vi "main.vi"() -> ()   [LabVIEW 2017]
uses:
  libraryGcode/ControlGlobal/stateModeDevice.ctl
  libraryGcode/control/stateBoardFirmware.ctl
  libraryGcode/control/Queue/QueueCMDandPOS.ctl
  libraryGcode/control/Queue/TypeDataPOS.ctl
  libraryGcode/control/stateCmdUpdatePara.ctl
  C:/Users/annha/Desktop/Inverse Kinematic - demo/controls/Robot_definition.ctl
  LIN3D/Robot_testing_instructions.ctl
  libraryGcode/control/TypeFirmwareControl.ctl
  libraryGcode/ClassStringGcode/XuLyDataDisplay.lvclass
  <vilib>/Platform/TimedLoop/XDataNode/timing_clust.ctl
  <vilib>/Platform/TimedLoop/XDataNode/nitl_modes.ctl
  <vilib>/Platform/TimedLoop/XDataNode/wakeup.ctl
  libraryGcode/ClassParameter/stateLoop_View.ctl
  libraryGcode/ClassStringGcode/SelectMcode.ctl
  libraryGcode/ClassStringGcode/SelectGcode.ctl
  libraryGcode/variableGlobal/StartAutoandGcode.vi
  <vilib>/Platform/TimedLoop/XDataNode/XDataNode.xnode
  libraryGcode/LibraryGcode.lvlib
  <vilib>/Platform/TimedLoop/XDataNode/XDNodeRunTimeDep.lvlib
  <vilib>/picture/3D Picture Control/NI_3D Picture Control.lvlib
  libraryGcode/ClassParameter/ParameterConf.lvclass
panel:
  out "logical OR":bool
  in  "LeapJog":cluster{"X":sgl, "Y":sgl, "Z":sgl}
  out "degrees":cluster{"A":dbl, "B":dbl}
  out "error out 2":errorcluster
  out "error out":errorcluster
  out "data GET":string="w\n"
  out "POS":cluster{"X":dbl, "Y":dbl, "Z":dbl}
  out "STATE BOARD":T1=enum."Waiting"
  out "statusMode":T2=enum."Menu"
  in  "SwitchMode":bool
  in  "Exit Program":bool=TRUE
  in  "Tab Control":enum32{"Setting", "Auto", "Config", ""}(tab)
  out "Boolean":bool
  out "G2-G3 PARA":cluster{"X":dbl, "Y":dbl, "I":dbl, "J":dbl}
  in  "Send Gcode manual":T3
  in  "BUTTON CONTROL GCODE FILE":T4={"FILE"={"AddFile_ButtonSaveFile"=FALSE, "AddFile_ButtonDeleteLastLine"=FALSE, "AddFile_ButtonDeleteAll"=FALSE}, "MOTION"={"AddFile_ButtonGoHome"=TRUE, "AddFile_ButtonAddG1"=FALSE, "AddFile_ButtonAddG0"=FALSE}}
  in  "BUTTON CONTROL MANUAL":T5
  in  "PARA":cluster{"STEP":i16, "FEEDRATE":dbl}={"STEP"=10, "FEEDRATE"=500.0} {"FEEDRATE" min=0.0 max=10000.0 step=50.0; "STEP" min=0 max=90 step=2 format="%-1.0f"}
  in  "CONTROL PWM":T6={"SPIN"={"PWM"=55.0, "Control_buttonSpindle"=FALSE, "ButtonSPINDLE_ADD_FILE"=FALSE}, "FAN 1"={"Control_ButtonFan1"=FALSE, "PWM"=255.0, "AddFile_ButtonFan1"=FALSE}, "FAN 2"={"PWM"=0.0, "Control_ButtonFan2"=FALSE, "AddFile_ButtonFan2"=FALSE}, "FAN 3"={"PWM"=0.0, "Control_ButtonFan3"=FALSE, "AddFile_ButtonFan3"=FALSE}, "WAIT PIN"={"PIN INPUT"=55.0, "Control_ButtonWaitPin"=FALSE, "AddFile_ButtonWaitPin"=FALSE}, "SOLENOID"={"Control_ButtonSolenoid"=FALSE, "AddFile_ButtonSolenoid"=FALSE}} {"WAIT PIN"."PIN INPUT" min=55.0 max=58.0 step=1.0; "FAN 3"."PWM" min=0.0 max=255.0 step=5.0; "FAN 2"."PWM" min=0.0 max=255.0 step=5.0; "FAN 1"."PWM" min=0.0 max=255.0 step=10.0; "SPIN"."PWM" min=0.0 max=255.0 step=1.0}
  in  "Link Save File":path
  out "GCODE ADD":string="\r"
  in  "File to Cut":path
  in  "Start Auto":bool
  out "G-Code Array 2":string[](array[string])=["Loi khong ket noChua Chon File"]
  in  "RESET ERROR":bool
  in  "MAX FEEDRATE":T7={"DATA"={"X"=4000.0, "Y"=4000.0, "Z"=4000.0}, "Config_SetFeedrate"=FALSE}
  in  "MAX ACCEL":T8={"DATA"={"X"=5000.0, "Y"=5000.0, "Z"=500.0}, "Config_SetMaxACCEL"=FALSE}
  in  "STEPSIZE":T9={"DATA"={"X"=88.89, "Y"=88.89, "Z"=2133.33}, "Config_SetStepSize"=FALSE}
  in  "M204 Start AcceL":T10={"Config_SetSTARTACCEL"=FALSE, "data"={"P"=88.89, "R"=88.89, "T"=2133.33}}
  in  "Move":cluster{"X":dbl, "Y":dbl, "OK Button":bool}
  in  "Config_SaveEEPROM":bool
  out "output cluster 2":cluster{"angle 1":dbl, "angle 2":dbl, i32}
  out "3D Picture":refnum<vi>(3d-picture)
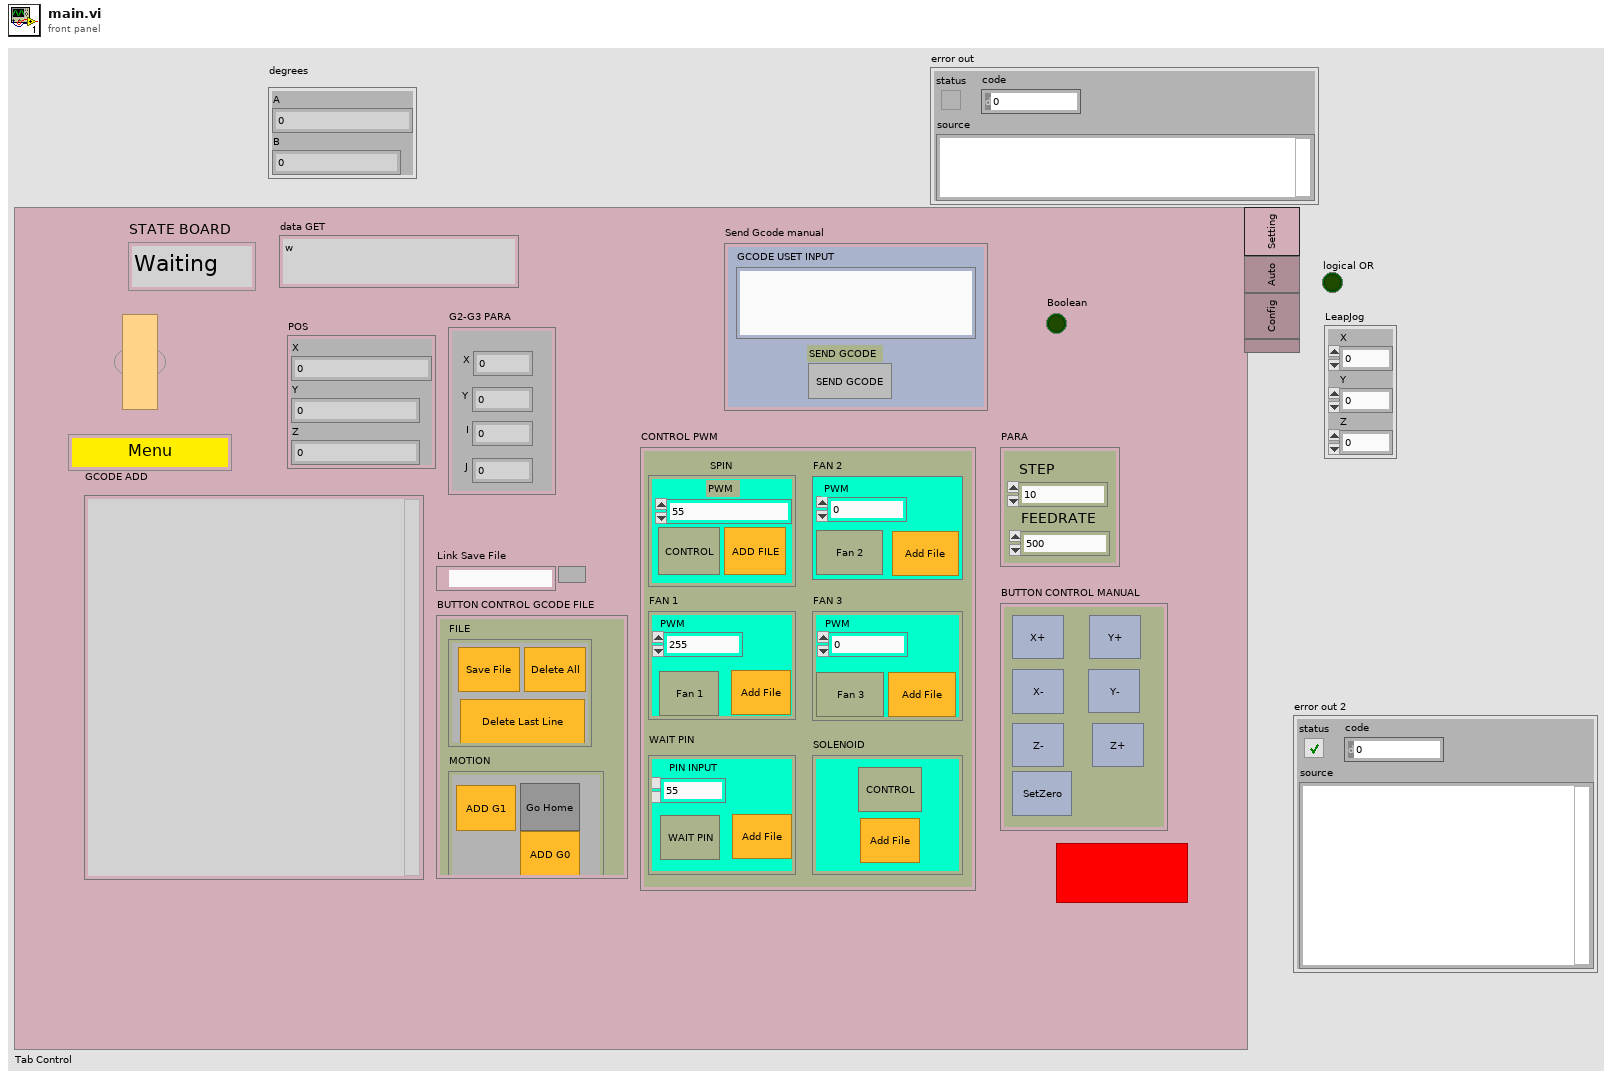
[diagram p1: front panel]
types:
  T1 = typedef "LibraryGcode.lvlib/stateBoardFirmware.ctl" = enum16{"Running", "Waiting", "Pos", "IDLE"}
  T2 = typedef "stateModeDevice.ctl" = enum16{"Auto", "Menu", "WaitAutoFinish", "Config", "initAuto"}
  T3 = cluster{"GCODE USET INPUT":string, "SEND GCODE":bool}
  T4 = cluster{"FILE":cluster{"AddFile_ButtonSaveFile":bool, "AddFile_ButtonDeleteLastLine":bool, "AddFile_ButtonDeleteAll":bool}, "MOTION":cluster{"AddFile_ButtonGoHome":bool, "AddFile_ButtonAddG1":bool, "AddFile_ButtonAddG0":bool}}
  T5 = cluster{"Control_ButtonX+":bool, "Control_ButtonX-":bool, "Control_ButtonY+":bool, "Control_ButtonY-":bool, "Control_ButtonZ+":bool, "Control_ButtonZ-":bool, "Control_ButtonSetZero":bool}
  T6 = cluster{"SPIN":cluster{"PWM":dbl, "Control_buttonSpindle":bool, "ButtonSPINDLE_ADD_FILE":bool}, "FAN 1":cluster{"Control_ButtonFan1":bool, "PWM":dbl, "AddFile_ButtonFan1":bool}, "FAN 2":cluster{"PWM":dbl, "Control_ButtonFan2":bool, "AddFile_ButtonFan2":bool}, "FAN 3":cluster{"PWM":dbl, "Control_ButtonFan3":bool, "AddFile_ButtonFan3":bool}, "WAIT PIN":cluster{"PIN INPUT":dbl, "Control_ButtonWaitPin":bool, "AddFile_ButtonWaitPin":bool}, "SOLENOID":cluster{"Control_ButtonSolenoid":bool, "AddFile_ButtonSolenoid":bool}}
  T7 = cluster{"DATA":cluster{"X":dbl, "Y":dbl, "Z":dbl}, "Config_SetFeedrate":bool}
  T8 = cluster{"DATA":cluster{"X":dbl, "Y":dbl, "Z":dbl}, "Config_SetMaxACCEL":bool}
  T9 = cluster{"DATA":cluster{"X":dbl, "Y":dbl, "Z":dbl}, "Config_SetStepSize":bool}
  T10 = cluster{"Config_SetSTARTACCEL":bool, "data":cluster{"P":dbl, "R":dbl, "T":dbl}}
  T11 = typedef "Robot_testing_instructions.ctl" = enum16{"idle", "Draw Robot", "Init 1 - Application", "Quit", "Close", "Error Handling", "Calculates"}
  T12 = typedef "Robot_definition.ctl" = cluster{"L2":sgl, "L3":sgl, "L1":sgl, "Base":sgl, "X0":sgl, "Z0":sgl}
  T13 = cluster{"Scene ref":refnum<vi>, "Arm 1 ref":refnum<vi>, "Arm 2 ref":refnum<vi>, "Arm 1 offset":cluster{"X":sgl, "Y":sgl, "Z":sgl}[], "Arm 2 offset":cluster{"X":sgl, "Y":sgl, "Z":sgl}[], "sand box":refnum<vi>, "Status":string, "A1":dbl, "A2":dbl, "Robot Definition":T12}
  T14 = typedef "LibraryGcode.lvlib/stateCmdUpdatePara.ctl" = enum16{"updatePos", "UpdateConfigAccel", "UpdateConfigFeed", "UpdateConfigUnit", "UpdateConfigStartAccel", "NoUpdate"}
  T15 = cluster{"Command":T14, "POS":cluster{"X":dbl, "Y":dbl, "Z":dbl}, "DEGREES":cluster{"X":dbl, "Y":dbl}}
  T16 = typedef "LibraryGcode.lvlib/QueueCMDandPOS.ctl" = cluster{"Serial Data Gcode":refnum<queue>, "cmdUpdateDisplay":refnum<queue>}
  T17 = typedef "LibraryGcode.lvlib/TypeFirmwareControl.ctl" = enum16{"ScaraMarlin", "CncMarlin", "Mk4Due"}
  T18 = typedef "XDNodeRunTimeDep.lvlib/timing_clust.ctl" = cluster{"Expected End [f-1]":u64, "Actual End [f-1]":u64, "Finished Late? [f-1]":bool, "Expected End [i-1]":u64, "Actual End [i-1]":u64, "Finished Late? [i-1]":bool, "Expected Start [i]":u64, "Actual Start [i]":u64, "Expected Start [f]":u64, "Actual Start [f]":u64, "Source Name":string, "Structure Name":string, "Period":i64, "Deadline":i64, "Offset":i64, "Start":i64, "Priority":i32, "Timeout":i32, "Mode":T19, "Wakeup Reason":T20, "Error":errorcluster, "Source Type":string, "Secondary Source Type":string, "Global End Time":u64, "Global Start Time":u64, "Frame Duration":u64, "Iteration Duration":u64, "Assigned CPU":i32, "I/O Scan Engine Mode":u32}
  T19 = typedef "XDNodeRunTimeDep.lvlib/nitl_modes.ctl" = enum32{"No Change", "Process missed periods, maintain original phase", "Discard missed periods, maintain original phase", "Process missed periods, ignore original phase", "Discard missed periods, ignore original phase"}
  T20 = typedef "XDNodeRunTimeDep.lvlib/wakeup.ctl" = enum32{"Normal", "Aborted", "Asynchronous wakeup", "Timing source error", "Timed loop error", "Timeout"}
  T21 = typedef "LibraryGcode.lvlib/XuLyDataDisplay.lvclass/SelectMcode.ctl" = enum16{"M204_SetStartingAcceleration", "M503_ReportSetting", "M500_SaveEprom", "M114_GetPosition", "M92_SetAxisStepPerUnit", "M17_EnableStep", "M18_DisableStep", "M80_PowerOn", "M81_PowerOff", "M112_EMGStop", "M118_SerialPrint", "M226_WaitforPinState", "M400_WaitFinishMove", "M203_SetMaxFeedRate", "M201_SetMaxACCEL", "M380_381_SetSoleNoid_On_Off", "M42_InitPin", "M42_PinControl", "M106_SetFan1", "M106_SetFan2", "M106_SetFan3", "M3_SetSpindle", "M5_OffSpindle", "M999_RestartStop"}
  T22 = typedef "LibraryGcode.lvlib/ParameterConf.lvclass/stateLoop_View.ctl" = enum16{"Running", "writeGlobal", "schedules500ms", "init", "End"}
  T23 = enum16{"Fan1", "Fan2", "Fan3", "PARA", "POS_DEGREE", "Solenoid", "Spindle", "TypeFirmware", "WaitPin", "MaxAcel", "MaxFeedrate", "MaxSize", "MaxStartAccel"}
  T24 = typedef "LibraryGcode.lvlib/XuLyDataDisplay.lvclass/SelectGcode.ctl" = enum16{"G0LinearMove", "G1XY", "G1LinearMove", "G2Arc", "G4Dwell", "G20InchUnit", "G21MilliUnit", "G28AutoHome", "G92SetPosition", "G90", "G91RelativePos", "JogX+", "JogX-", "JogY+", "JogY-", "JogZ+", "JogZ-", "sendGcodeString"}
  T25 = cluster{"SPIN":dbl, "FAN2":dbl, "FAN1":dbl, "FAN3":dbl, "WAIT PIN ":dbl}
  T26 = cluster{"PWM":dbl, "TypeFirmware":T17, "XYZ":cluster{"X":dbl, "Y":dbl, "Z":dbl}, "PARA":cluster{"STEP":i16, "FEEDRATE":dbl}, "DEGREES":cluster{"X":dbl, "Y":dbl}, "Solenoid":bool, "StartAccel":cluster{"P":dbl, "R":dbl, "T":dbl}}
  T27 = typedef "Robot_creation_loop_data.ctl" = cluster{"Robot Definition":T12, "Dispenser ref":refnum<vi>, "Arm 2 ref":refnum<vi>, "Arm 1 ref":refnum<vi>, "Base ref":refnum<vi>, "Scene ref":refnum<vi>, "Sand box ref":refnum<vi>, "Arm 1 Offset":cluster{"X":sgl, "Y":sgl, "Z":sgl}[], "Arm 2 Offset":cluster{"X":sgl, "Y":sgl, "Z":sgl}[], "Width":sgl}
  T28 = cluster{"error out":errorcluster, "error IO 2":errorcluster}
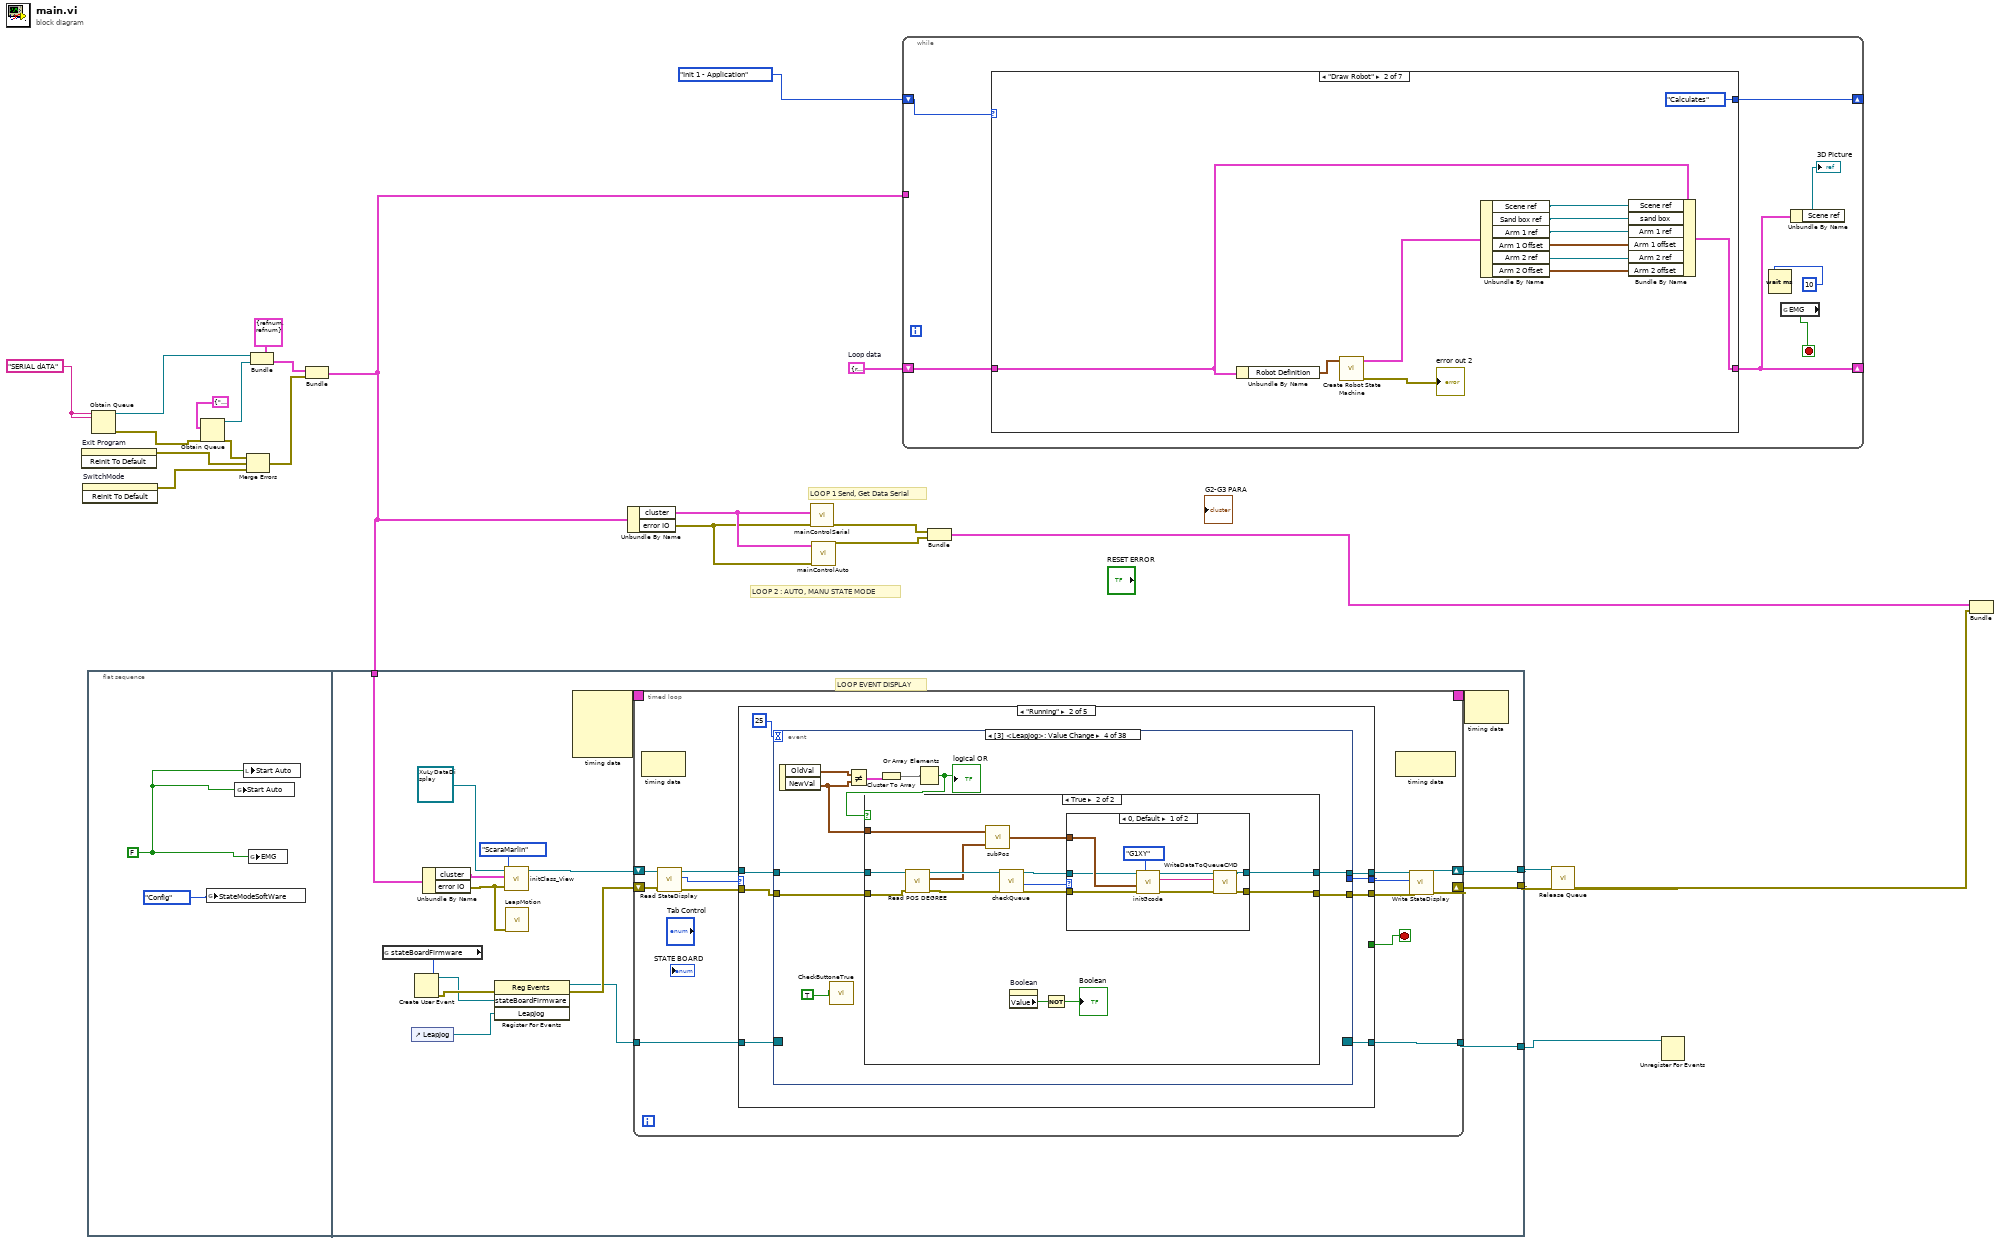
[diagram p0: block diagram]
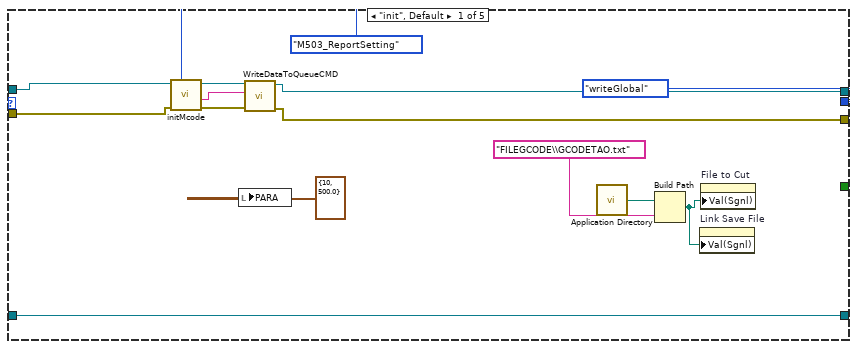
[diagram p2: hidden frame]
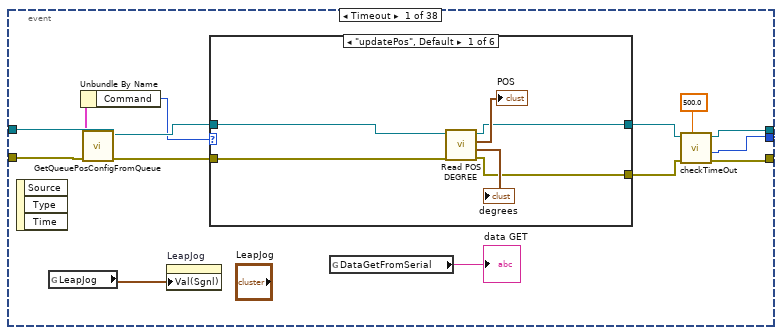
[diagram p3: hidden frame]
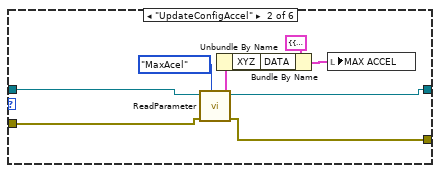
[diagram p4: hidden frame]
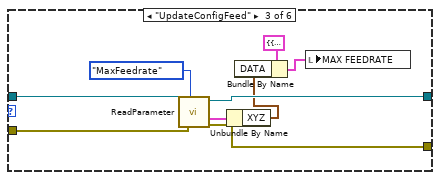
[diagram p5: hidden frame]
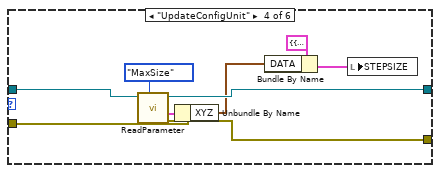
[diagram p6: hidden frame]
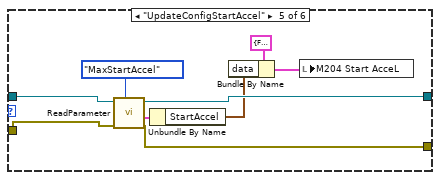
[diagram p7: hidden frame]
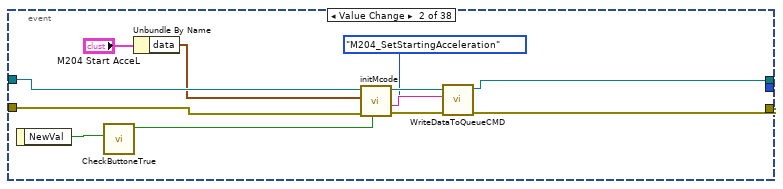
[diagram p9: hidden frame]
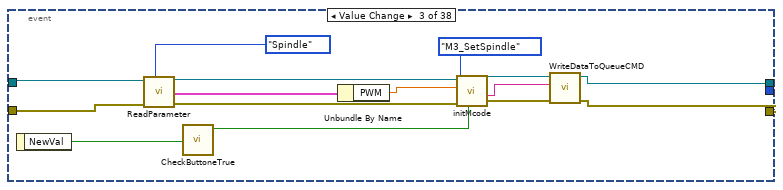
[diagram p10: hidden frame]
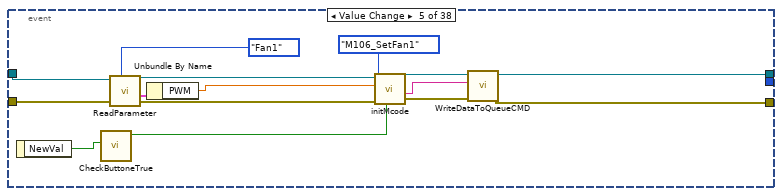
[diagram p13: hidden frame]
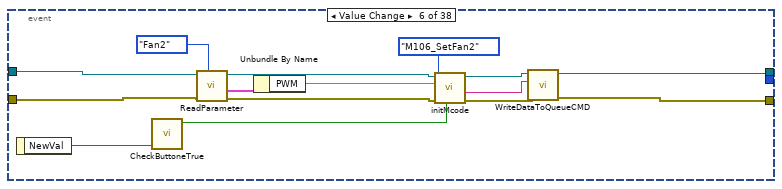
[diagram p14: hidden frame]
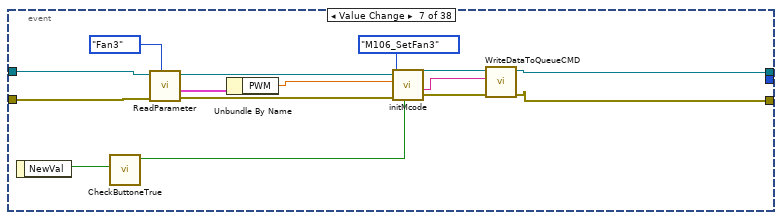
[diagram p15: hidden frame]
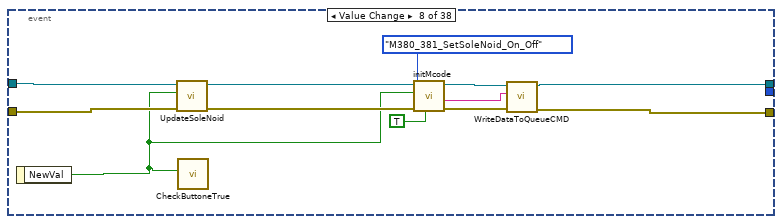
[diagram p16: hidden frame]
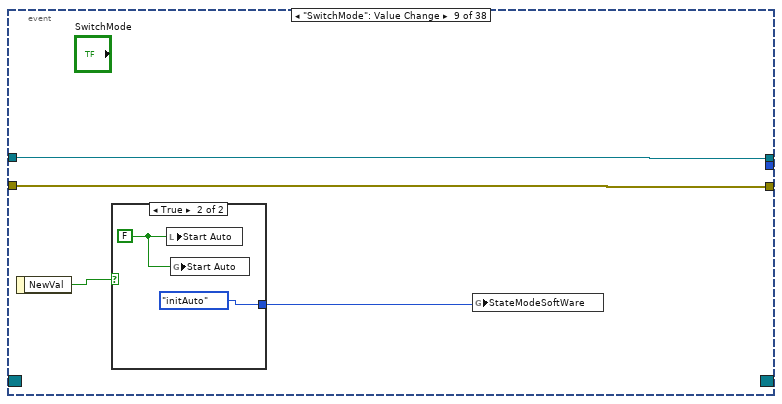
[diagram p17: hidden frame]
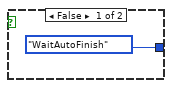
[diagram p18: hidden frame]
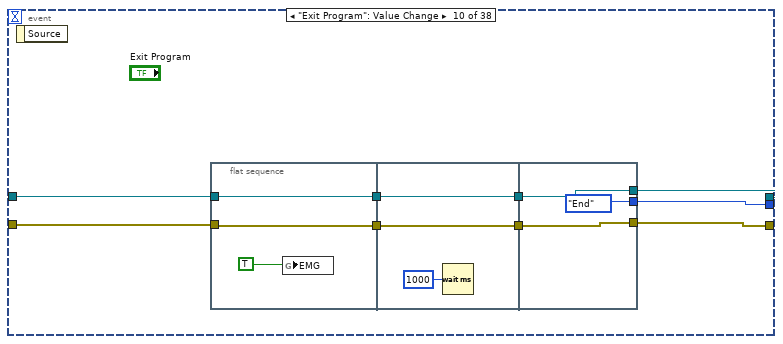
[diagram p19: hidden frame]
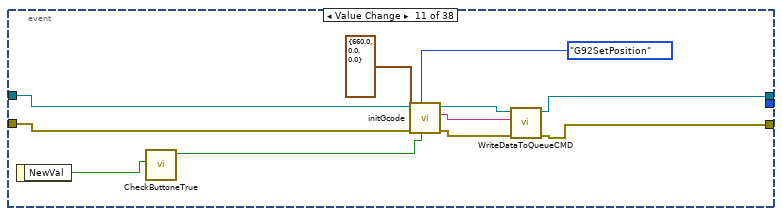
[diagram p20: hidden frame]
diagram:
  w9 = T13 {"Scene ref"=refnum, "Arm 1 ref"=refnum, "Arm 2 ref"=refnum, "Arm 1 offset"=[], "Arm 2 offset"=[], "sand box"=refnum, "Status"="", "A1"=43.0, "A2"=23.0, "Robot Definition"={"L2"=0.0, "L3"=0.0, "L1"=0.0, "Base"=0.0, "X0"=0.0, "Z0"=0.0}}  # Loop data
  w23 = "SERIAL dATA" ("name (unnamed)")
  # "LOOP 2 : AUTO, MANU STATE MODE"
  # "LOOP 1 Send, Get Data Serial"
  n1 = invoke on="Exit Program" class="Bool (strict)" method="Reinit To Default"() -> (error out=w21:errorcluster)  [unwired: 3 in, 2 out]
  n2 = invoke on="SwitchMode" class="Bool (strict)" method="Reinit To Default"() -> (error out=w22:errorcluster)  [unwired: 3 in, 2 out]
  n3 = flat-sequence {
    tunnel: [w42] -> w3
    tunnel: w11 -> [w41]
    tunnel: [w38] -> w4
    tunnel: [w28] -> w1
    frame #0 {
      w25 = FALSE ("Start Auto")
      n4 = global write "StartAutoandGcode.vi" "StateModeSoftWare"(stateModeDevice."Config" ("Enum")) -> ()
      n5 = global write "StartAutoandGcode.vi" "Start Auto"(w25) -> ()
      n6 = local write "Start Auto"(w25) -> ()
      n7 = global write "StartAutoandGcode.vi" "EMG"(w25) -> ()
    }
    frame #1 {
      # "LOOP EVENT DISPLAY"
      n8 = global read "StartAutoandGcode.vi" "stateBoardFirmware"() -> (w30:T1)
      n9 = control-ref of="LeapJog"() -> (w27:refnum<vi>)
      n10 = Create User Event(user event datatype=w30) -> (user event=w29:refnum<user-event>, error out=w32:errorcluster)  [unwired: 1 in]
      n11 = Unbundle By Name(w41) -> ("cluster"=w37:T16, "error IO"=w26:errorcluster)
      n12 = register-events(error in=w32, w29, w27) -> (reference out=w31:refnum<event-registration>, error out=w33:errorcluster)  [unwired: 1 in]
      n13 = call-dynamic "initClass_View.vi"("error in (no error)"=w26, "TypeFirmware"=TypeFirmwareControl."ScaraMarlin", "Queue Process"=w37, "XuLyDataDisplay in"=refnum<class "XuLyDataDisplay.lvclass"> refnum) -> ("XuLyDataDisplay out"=w35:refnum<class "XuLyDataDisplay.lvclass">)  [unwired: 6 in, 1 out]
      n14 = call "LeapMotion.vi"("Error In"=w26) -> ()  [unwired: 9 in, 2 out]
      n15 = node-c288() -> (w40:T18)  [unwired: 4 in]
      n16 = timed-loop {
        timing: w40 -> [_]
        timing-out: [_] -> w39
        shift-right: [w50] -> w38
        shift-left: w35 -> [w54]
        shift-right: [w49] -> w42
        shift-left: w33 -> [w52]
        tunnel: w31 -> [w44]
        tunnel: [w43] -> w28
        stop <- w55 stop-if-true
        n17 = node-c288() -> ()  [unwired: 1 in, 1 out]
        n18 = call-dynamic "Read StateDisplay.vi"("error in (no error)"=w52, "ParameterConf in"=w54) -> ("error out"=w51:errorcluster, "StateDisplay"=w47:T22, "ParameterConf out"=w53:refnum<class "XuLyDataDisplay.lvclass">)  [unwired: 7 in]
        n19 = case shown="\"Running\"" w47 {
          tunnel: w51 -> [w62 w72 w580 w592 w609]
          tunnel: [_ _ TRUE _ _] -> w55
          tunnel: [w61 w76 w580 w590 w606] -> w48
          tunnel: w53 -> [w66 w78 w579 w593 w610]
          tunnel: [w63 w74 w579 w591 w607] -> w45
          tunnel: [stateLoop_View."writeGlobal" ("StateDisplay") w77 stateLoop_View."init" ("StateDisplay") stateLoop_View."schedules500ms" ("StateDisplay") stateLoop_View."Running" ("StateDisplay")] -> w46
          tunnel: w44 -> [w58 w75 w577 w582 w604]
          tunnel: [w58 w73 w577 w582 w604] -> w43
          frame "init", Default {
            n20 = call-dynamic "initMcode.vi"("error in (no error)"=w62, "mCode"=SelectMcode."M503_ReportSetting", "XuLyDataDisplay in"=w66) -> ("error out"=w60:errorcluster, "McodeOut"=w64:string, "XuLyDataDisplay out"=w65:refnum<class "XuLyDataDisplay.lvclass">)  [unwired: 6 in]
            n21 = local write "PARA"(cluster{"STEP":i16, "FEEDRATE":dbl} {"STEP"=10, "FEEDRATE"=500.0} ("PARA")) -> ()
            n22 = call-dynamic "WriteDataToQueueCMD.vi"("error in (no error)"=w60, "DataIn"=w64, "ParameterConf in"=w65) -> ("error out"=w61:errorcluster, "ParameterConf out"=w63:refnum<class "XuLyDataDisplay.lvclass">)  [unwired: 7 in]
            n23 = call <vilib>:"Application Directory.vi"() -> ("Application Directory"=w69:path)
            n24 = Build Path(base path=w69, name or relative path="FILEGCODE\\GCODETAO.txt") -> (appended path=w71:path)
            n25 = property on="Link Save File" class="Path"("Val(Sgnl)"=w71) -> ()  [unwired: 2 in, 2 out]
            n26 = property on="File to Cut" class="Path"("Val(Sgnl)"=w71) -> ()  [unwired: 2 in, 2 out]
          }
          frame "Running" {
            n27 = event shown="[3] <LeapJog>: Value Change" {
              selector: w75 -> [_ _ _ _ _ _ _ _ _ _ _ _ _ _ _ _ _ _ _ _ _ _ _ _ _ _ _ _ _ _ _ _ _ _ w536 _ _ _]
              dyn-events: [_ _ _ _ _ _ _ _ _ _ _ _ _ _ _ _ _ _ _ _ _ _ _ _ _ _ _ _ _ _ _ _ _ _ w536 _ _ _] -> w73
              timeout: 25 -> [_ _ _ _ _ _ _ _ _ _ _ _ _ _ _ _ _ _ _ _ _ _ _ _ _ _ _ _ _ _ _ _ _ _ _ _ _ _]
              tunnel: w72 -> [w92 w142 w162 w168 w213 w228 w244 w256 w261 w267 w290 w295 w300 w312 w328 w337 w351 w364 w370 w382 w395 w401 w420 w435 w446 w463 w478 w484 w488 w490 w499 w511 w521 w533 w544 w554 w560 w570]
              tunnel: [w84 w145 w153 w167 w209 w222 w238 w250 w261 w266 w285 w295 w298 w314 w323 w339 w348 w359 w370 w374 w395 w400 w407 w423 w438 w453 w466 w481 w488 w491 w502 w505 w522 w531 w540 w547 w557 w569] -> w76
              tunnel: w78 -> [w93 w148 w163 w170 w214 w229 w243 w257 w260 w270 w291 w294 w301 w316 w329 w342 w352 w366 w369 w383 w396 w402 w421 w436 w447 w464 w479 w485 w487 w493 w501 w512 w524 w534 w545 w555 w561 w571]
              tunnel: [w85 w146 w154 w169 w210 w223 w239 w253 w260 w273 w286 w294 w296 w313 w324 w340 w349 w357 w369 w373 w396 w397 w408 w424 w439 w454 w467 w482 w487 w489 w494 w506 w523 w532 w541 w548 w558 w567] -> w74
              tunnel: [w82 _ _ _ _ _ _ _ _ w265 _ _ _ _ _ _ _ _ _ _ stateLoop_View."writeGlobal" ("StateDisplay") _ _ _ _ _ _ _ _ _ _ _ _ _ _ _ _ _] -> w77
              event Timeout {
                n28 = event-data() -> ()  [unwired: 1 in, 3 out]
                n29 = global read "StartAutoandGcode.vi" "LeapJog"() -> (w80:cluster{"X":sgl, "Y":sgl, "Z":sgl})
                n30 = call-dynamic "GetQueuePosConfigFromQueue.vi"("error in (no error)"=w92, "ParameterConf in"=w93) -> ("error out"=w89:errorcluster, "element"=w91:T15, "ParameterConf out"=w90:refnum<class "XuLyDataDisplay.lvclass">)  [unwired: 7 in]
                n31 = Unbundle By Name(w91) -> ("Command"=w81:T14)
                n32 = property on="LeapJog" class="Clust (strict)"("Val(Sgnl)"=w80) -> ()  [unwired: 2 in, 2 out]
                n33 = case shown="\"updatePos\", Default" w81 {
                  tunnel: [w95 w108 w115 w125 w134 w137] -> w87
                  tunnel: w90 -> [w97 w107 w117 w118 w130 w137]
                  tunnel: [w94 w105 w114 w124 w133 w136] -> w86
                  tunnel: w89 -> [w96 w106 w116 w126 w135 w136]
                  frame "updatePos", Default {
                    n34 = call-dynamic "Read POS DEGREE.vi"("error in (no error)"=w96, "ParameterConf in"=w97) -> ("error out"=w94:errorcluster, "DEGREES"=→"degrees":cluster{"X":dbl, "Y":dbl}, "POS"=→"POS":cluster{"X":dbl, "Y":dbl, "Z":dbl}, "ParameterConf out"=w95:refnum<class "XuLyDataDisplay.lvclass">)  [unwired: 6 in]
                  }
                  frame "UpdateConfigAccel" {
                    n35 = call-dynamic "ReadParameter.vi"("ParameterConf in"=w107, "error in (no error)"=w106, "Parameter"=T23."MaxAcel") -> ("ParameterConf out"=w108:refnum<class "XuLyDataDisplay.lvclass">, "DataOutClust"=w101:T26, "error out"=w105:errorcluster)  [unwired: 4 in, 1 out]
                    n36 = Unbundle By Name(w101) -> ("XYZ"=w100:cluster{"X":dbl, "Y":dbl, "Z":dbl})
                    n37 = Bundle By Name(cluster=T8 {"DATA"={"X"=355.0, "Y"=355.0, "Z"=2133.0}, "Config_SetMaxACCEL"=FALSE} ("MAX ACCEL"), "DATA"=w100) -> (w103:T8)
                    n38 = local write "MAX ACCEL"(w103) -> ()
                  }
                  frame "UpdateConfigFeed" {
                    n39 = call-dynamic "ReadParameter.vi"("ParameterConf in"=w117, "error in (no error)"=w116, "Parameter"=T23."MaxFeedrate") -> ("ParameterConf out"=w115:refnum<class "XuLyDataDisplay.lvclass">, "DataOutClust"=w110:T26, "error out"=w114:errorcluster)  [unwired: 4 in, 1 out]
                    n40 = Unbundle By Name(w110) -> ("XYZ"=w109:cluster{"X":dbl, "Y":dbl, "Z":dbl})
                    n41 = Bundle By Name(cluster=T9 {"DATA"={"X"=355.56, "Y"=355.56, "Z"=2133.33}, "Config_SetStepSize"=FALSE} ("STEPSIZE"), "DATA"=w109) -> (w112:T9)
                    n42 = local write "MAX FEEDRATE"(w112) -> ()
                  }
                  frame "UpdateConfigUnit" {
                    n43 = call-dynamic "ReadParameter.vi"("ParameterConf in"=w118, "error in (no error)"=w126, "Parameter"=T23."MaxSize") -> ("ParameterConf out"=w125:refnum<class "XuLyDataDisplay.lvclass">, "DataOutClust"=w120:T26, "error out"=w124:errorcluster)  [unwired: 4 in, 1 out]
                    n44 = Unbundle By Name(w120) -> ("XYZ"=w119:cluster{"X":dbl, "Y":dbl, "Z":dbl})
                    n45 = Bundle By Name(cluster=T7 {"DATA"={"X"=150000.0, "Y"=150000.0, "Z"=10000.0}, "Config_SetFeedrate"=FALSE} ("MAX FEEDRATE"), "DATA"=w119) -> (w122:T7)
                    n46 = local write "STEPSIZE"(w122) -> ()
                  }
                  frame "UpdateConfigStartAccel" {
                    n47 = call-dynamic "ReadParameter.vi"("ParameterConf in"=w130, "error in (no error)"=w135, "Parameter"=T23."MaxStartAccel") -> ("ParameterConf out"=w134:refnum<class "XuLyDataDisplay.lvclass">, "DataOutClust"=w128:T26, "error out"=w133:errorcluster)  [unwired: 4 in, 1 out]
                    n48 = Unbundle By Name(w128) -> ("StartAccel"=w127:cluster{"P":dbl, "R":dbl, "T":dbl})
                    n49 = Bundle By Name(cluster=T10 {"Config_SetSTARTACCEL"=FALSE, "data"={"P"=355.56, "R"=355.56, "T"=2133.33}} ("M204 Start AcceL"), "data"=w127) -> (w131:T10)
                    n50 = local write "M204 Start AcceL"(w131) -> ()
                  }
                  frame "NoUpdate" {
                  }
                }
                n51 = global read "StartAutoandGcode.vi" "DataGetFromSerial"() -> (→"data GET":string)
                n52 = call-dynamic "checkTimeOut.vi"("error in (no error)"=w86, "Time"=500.0, "ParameterConf in"=w87) -> ("error out"=w84:errorcluster, "stateDisplay"=w82:T22, "ParameterConf out"=w85:refnum<class "XuLyDataDisplay.lvclass">)  [unwired: 5 in, 1 out]
              }
              event "M204 Start AcceL.Config_SetSTARTACCEL": Value Change {
                n53 = event-data() -> ("NewVal"=w149:bool)  [unwired: 1 in]
                n54 = call "CheckButtoneTrue.vi"("IN"=w149) -> ("OUT"=w138:bool)  [unwired: 10 in]
                n55 = Unbundle By Name("M204 Start AcceL") -> ("data"=w140:cluster{"P":dbl, "R":dbl, "T":dbl})
                n56 = call-dynamic "initMcode.vi"("CheckMenu"=w138, "error in (no error)"=w142, "mCode"=SelectMcode."M204_SetStartingAcceleration", "DataVariant"=w140, "XuLyDataDisplay in"=w148) -> ("error out"=w144:errorcluster, "McodeOut"=w143:string, "XuLyDataDisplay out"=w147:refnum<class "XuLyDataDisplay.lvclass">)  [unwired: 4 in]
                n57 = call-dynamic "WriteDataToQueueCMD.vi"("error in (no error)"=w144, "DataIn"=w143, "ParameterConf in"=w147) -> ("error out"=w145:errorcluster, "ParameterConf out"=w146:refnum<class "XuLyDataDisplay.lvclass">)  [unwired: 7 in]
              }
              event "CONTROL PWM.SPIN.Control_buttonSpindle": Value Change {
                n58 = event-data() -> ("NewVal"=w164:bool)  [unwired: 1 in]
                n59 = call-dynamic "ReadParameter.vi"("ParameterConf in"=w163, "error in (no error)"=w162, "Parameter"=T23."Spindle") -> ("ParameterConf out"=w160:refnum<class "XuLyDataDisplay.lvclass">, "DataOutClust"=w152:T26, "error out"=w159:errorcluster)  [unwired: 4 in, 1 out]
                n60 = call "CheckButtoneTrue.vi"("IN"=w164) -> ("OUT"=w157:bool)  [unwired: 10 in]
                n61 = Unbundle By Name(w152) -> ("PWM"=w151:dbl)
                n62 = call-dynamic "initMcode.vi"("CheckMenu"=w157, "error in (no error)"=w159, "mCode"=SelectMcode."M3_SetSpindle", "DataVariant"=w151, "XuLyDataDisplay in"=w160) -> ("error out"=w158:errorcluster, "McodeOut"=w156:string, "XuLyDataDisplay out"=w161:refnum<class "XuLyDataDisplay.lvclass">)  [unwired: 4 in]
                n63 = call-dynamic "WriteDataToQueueCMD.vi"("error in (no error)"=w158, "DataIn"=w156, "ParameterConf in"=w161) -> ("error out"=w153:errorcluster, "ParameterConf out"=w154:refnum<class "XuLyDataDisplay.lvclass">)  [unwired: 7 in]
              }
              event Value Change {
                n64 = event-data() -> ("OldVal"=w173:cluster{"X":sgl, "Y":sgl, "Z":sgl}, "NewVal"=w165:cluster{"X":sgl, "Y":sgl, "Z":sgl})  [unwired: 1 in]
                n65 = call "CheckButtoneTrue.vi"("IN"=TRUE) -> ()  [unwired: 10 in, 1 out]
                n66 = Not Equal?(x=w173, y=w165) -> (x != y?=w172:cluster{"X":bool, "Y":bool, "Z":bool})
                n67 = Cluster To Array(cluster=w172) -> (array=w171:bool[])
                n68 = Or Array Elements(Boolean array=w171) -> (logical OR=w166:bool)
                "logical OR" <- w166
                n69 = case shown="True" w166 {
                  tunnel: w170 -> [w176 w189]
                  tunnel: [w176 w182] -> w169
                  tunnel: w168 -> [w175 w187]
                  tunnel: [w175 w181] -> w167
                  tunnel: w165 -> [_ w185]
                  frame False {
                  }
                  frame True {
                    n70 = call-dynamic "Read POS DEGREE.vi"("error in (no error)"=w187, "ParameterConf in"=w189) -> ("error out"=w183:errorcluster, "POS"=w186:cluster{"X":dbl, "Y":dbl, "Z":dbl}, "ParameterConf out"=w188:refnum<class "XuLyDataDisplay.lvclass">)  [unwired: 6 in, 1 out]
                    n71 = call "subPos.vi"("POS"=w186, "NewVal"=w185) -> ("PosSetG92"=w184:cluster{"X":dbl, "Y":dbl, "Z":dbl})
                    n72 = call-dynamic "checkQueue.vi"("ParameterConf in"=w188) -> ("Numeric"=w177:i16, "ParameterConf out"=w178:refnum<class "XuLyDataDisplay.lvclass">)  [unwired: 8 in, 1 out]
                    n73 = property on="Boolean" class="Bool (strict)"() -> ("Value"=w179:bool)  [unwired: 2 in, 2 out]
                    n74 = Not(x=w179) -> (.not. x?=→"Boolean":bool)
                    n75 = case shown="0, Default" w177 {
                      tunnel: w184 -> [w196 _]
                      tunnel: w183 -> [w195 w199]
                      tunnel: [w194 w200] -> w182
                      tunnel: [w191 w199] -> w181
                      tunnel: w178 -> [w190 w200]
                      frame 0, Default {
                        n76 = call-dynamic "initGcode.vi"("gCode"=SelectGcode."G1XY", "error in (no error)"=w195, "PosSetG92"=w196, "XuLyDataDisplay in"=w190) -> ("error out"=w192:errorcluster, "GcodeString Out"=w193:string, "XuLyDataDisplay out"=w198:refnum<class "XuLyDataDisplay.lvclass">)  [unwired: 5 in]
                        n77 = call-dynamic "WriteDataToQueueCMD.vi"("error in (no error)"=w192, "DataIn"=w193, "ParameterConf in"=w198) -> ("error out"=w191:errorcluster, "ParameterConf out"=w194:refnum<class "XuLyDataDisplay.lvclass">)  [unwired: 7 in]
                      }
                      frame 1 {
                      }
                    }
                  }
                }
              }
              event "CONTROL PWM.FAN 1.Control_ButtonFan1": Value Change {
                n78 = event-data() -> ("NewVal"=w215:bool)  [unwired: 1 in]
                n79 = call "CheckButtoneTrue.vi"("IN"=w215) -> ("OUT"=w204:bool)  [unwired: 10 in]
                n80 = call-dynamic "ReadParameter.vi"("ParameterConf in"=w214, "error in (no error)"=w213, "Parameter"=T23."Fan1") -> ("ParameterConf out"=w212:refnum<class "XuLyDataDisplay.lvclass">, "DataOutClust"=w203:T26, "error out"=w208:errorcluster)  [unwired: 4 in, 1 out]
                n81 = Unbundle By Name(w203) -> ("PWM"=w202:dbl)
                n82 = call-dynamic "initMcode.vi"("CheckMenu"=w204, "error in (no error)"=w208, "mCode"=SelectMcode."M106_SetFan1", "DataVariant"=w202, "XuLyDataDisplay in"=w212) -> ("error out"=w206:errorcluster, "McodeOut"=w205:string, "XuLyDataDisplay out"=w211:refnum<class "XuLyDataDisplay.lvclass">)  [unwired: 4 in]
                n83 = call-dynamic "WriteDataToQueueCMD.vi"("error in (no error)"=w206, "DataIn"=w205, "ParameterConf in"=w211) -> ("error out"=w209:errorcluster, "ParameterConf out"=w210:refnum<class "XuLyDataDisplay.lvclass">)  [unwired: 7 in]
              }
              event "CONTROL PWM.FAN 2.Control_ButtonFan2": Value Change {
                n84 = event-data() -> ("NewVal"=w230:bool)  [unwired: 1 in]
                n85 = call "CheckButtoneTrue.vi"("IN"=w230) -> ("OUT"=w220:bool)  [unwired: 10 in]
                n86 = call-dynamic "ReadParameter.vi"("ParameterConf in"=w229, "error in (no error)"=w228, "Parameter"=T23."Fan2") -> ("ParameterConf out"=w227:refnum<class "XuLyDataDisplay.lvclass">, "DataOutClust"=w218:T26, "error out"=w221:errorcluster)  [unwired: 4 in, 1 out]
                n87 = Unbundle By Name(w218) -> ("PWM"=w216:dbl)
                n88 = call-dynamic "initMcode.vi"("CheckMenu"=w220, "error in (no error)"=w221, "mCode"=SelectMcode."M106_SetFan2", "DataVariant"=w216, "XuLyDataDisplay in"=w227) -> ("error out"=w224:errorcluster, "McodeOut"=w226:string, "XuLyDataDisplay out"=w225:refnum<class "XuLyDataDisplay.lvclass">)  [unwired: 4 in]
                n89 = call-dynamic "WriteDataToQueueCMD.vi"("error in (no error)"=w224, "DataIn"=w226, "ParameterConf in"=w225) -> ("error out"=w222:errorcluster, "ParameterConf out"=w223:refnum<class "XuLyDataDisplay.lvclass">)  [unwired: 7 in]
              }
              event "CONTROL PWM.FAN 3.Control_ButtonFan3": Value Change {
                n90 = event-data() -> ("NewVal"=w245:bool)  [unwired: 1 in]
                n91 = call "CheckButtoneTrue.vi"("IN"=w245) -> ("OUT"=w234:bool)  [unwired: 10 in]
                n92 = call-dynamic "ReadParameter.vi"("ParameterConf in"=w243, "error in (no error)"=w244, "Parameter"=T23."Fan3") -> ("ParameterConf out"=w242:refnum<class "XuLyDataDisplay.lvclass">, "DataOutClust"=w232:T26, "error out"=w236:errorcluster)  [unwired: 4 in, 1 out]
                n93 = Unbundle By Name(w232) -> ("PWM"=w231:dbl)
                n94 = call-dynamic "initMcode.vi"("CheckMenu"=w234, "error in (no error)"=w236, "mCode"=SelectMcode."M106_SetFan3", "DataVariant"=w231, "XuLyDataDisplay in"=w242) -> ("error out"=w237:errorcluster, "McodeOut"=w241:string, "XuLyDataDisplay out"=w240:refnum<class "XuLyDataDisplay.lvclass">)  [unwired: 4 in]
                n95 = call-dynamic "WriteDataToQueueCMD.vi"("error in (no error)"=w237, "DataIn"=w241, "ParameterConf in"=w240) -> ("error out"=w238:errorcluster, "ParameterConf out"=w239:refnum<class "XuLyDataDisplay.lvclass">)  [unwired: 7 in]
              }
              event "CONTROL PWM.SOLENOID.Control_ButtonSolenoid": Value Change {
                n96 = event-data() -> ("NewVal"=w247:bool)  [unwired: 1 in]
                n97 = call-dynamic "UpdateSoleNoid.vi"("error in (no error)"=w256, "Boolean"=w247, "ParameterConf in"=w257) -> ("error out"=w252:errorcluster, "ParameterConf out"=w255:refnum<class "XuLyDataDisplay.lvclass">)  [unwired: 7 in]
                n98 = call "CheckButtoneTrue.vi"("IN"=w247) -> ()  [unwired: 10 in, 1 out]
                n99 = call-dynamic "initMcode.vi"("CheckMenu"=TRUE, "error in (no error)"=w252, "mCode"=SelectMcode."M380_381_SetSoleNoid_On_Off", "DataVariant"=w247, "XuLyDataDisplay in"=w255) -> ("error out"=w251:errorcluster, "McodeOut"=w248:string, "XuLyDataDisplay out"=w254:refnum<class "XuLyDataDisplay.lvclass">)  [unwired: 4 in]
                n100 = call-dynamic "WriteDataToQueueCMD.vi"("error in (no error)"=w251, "DataIn"=w248, "ParameterConf in"=w254) -> ("error out"=w250:errorcluster, "ParameterConf out"=w253:refnum<class "XuLyDataDisplay.lvclass">)  [unwired: 7 in]
              }
              event "SwitchMode": Value Change {
                n101 = event-data() -> ("NewVal"=w259:bool)  [unwired: 1 in]
                n102 = case shown="True" w259 {
                  tunnel: [stateModeDevice."WaitAutoFinish" ("Enum") stateModeDevice."initAuto" ("Enum")] -> w258
                  frame False {
                  }
                  frame True {
                    w263 = FALSE ("Start Auto")
                    n103 = local write "Start Auto"(w263) -> ()
                    n104 = global write "StartAutoandGcode.vi" "Start Auto"(w263) -> ()
                  }
                }
                n105 = global write "StartAutoandGcode.vi" "StateModeSoftWare"(w258) -> ()
              }
              event "Exit Program": Value Change {
                n106 = event-data() -> ()  [unwired: 1 in, 1 out]
                n107 = flat-sequence {
                  tunnel: [w276] -> w271
                  tunnel: w270 -> [w276]
                  tunnel: [w275] -> w268
                  tunnel: w267 -> [w275]
                  tunnel: [w278] -> w272
                  tunnel: w271 -> [w278]
                  tunnel: [w277] -> w269
                  tunnel: w268 -> [w277]
                  tunnel: [w282] -> w273
                  tunnel: w272 -> [w282]
                  tunnel: [w281] -> w266
                  tunnel: w269 -> [w281]
                  tunnel: [stateLoop_View."End" ("StateDisplay")] -> w265
                  frame #0 {
                    n108 = global write "StartAutoandGcode.vi" "EMG"(TRUE ("EMG1")) -> ()
                  }
                  frame #1 {
                    n109 = Wait (ms)(milliseconds to wait=u32 1000) -> ()  [unwired: 1 out]
                  }
                  frame #2 {
                  }
                }
              }
              event "BUTTON CONTROL MANUAL.Control_ButtonSetZero": Value Change {
                n110 = event-data() -> ("NewVal"=w284:bool)  [unwired: 1 in]
                n111 = call "CheckButtoneTrue.vi"("IN"=w284) -> ("OUT"=w283:bool)  [unwired: 10 in]
                n112 = call-dynamic "initGcode.vi"("Che Do"=w283, "gCode"=SelectGcode."G92SetPosition", "error in (no error)"=w290, "PosSetG92"=cluster{"X":dbl, "Y":dbl, "Z":dbl} {"X"=660.0, "Y"=0.0, "Z"=0.0}, "XuLyDataDisplay in"=w291) -> ("error out"=w287:errorcluster, "GcodeString Out"=w288:string, "XuLyDataDisplay out"=w289:refnum<class "XuLyDataDisplay.lvclass">)  [unwired: 4 in]
                n113 = call-dynamic "WriteDataToQueueCMD.vi"("error in (no error)"=w287, "DataIn"=w288, "ParameterConf in"=w289) -> ("error out"=w285:errorcluster, "ParameterConf out"=w286:refnum<class "XuLyDataDisplay.lvclass">)  [unwired: 7 in]
              }
              event "Tab Control": Value Change {
                n114 = event-data() -> ()  [unwired: 1 in, 1 out]
              }
              event "BUTTON CONTROL MANUAL.Control_ButtonX+": Value Change {
                n115 = event-data() -> ("NewVal"=w305:bool)  [unwired: 1 in]
                n116 = call "CheckButtoneTrue.vi"("IN"=w305) -> ("OUT"=w299:bool)  [unwired: 10 in]
                n117 = call-dynamic "initGcode.vi"("Che Do"=w299, "gCode"=SelectGcode."JogX+", "error in (no error)"=w300, "XuLyDataDisplay in"=w301) -> ("error out"=w303:errorcluster, "GcodeString Out"=w297:string, "XuLyDataDisplay out"=w304:refnum<class "XuLyDataDisplay.lvclass">)  [unwired: 5 in]
                n118 = call-dynamic "WriteDataToQueueCMD.vi"("error in (no error)"=w303, "DataIn"=w297, "ParameterConf in"=w304) -> ("error out"=w298:errorcluster, "ParameterConf out"=w296:refnum<class "XuLyDataDisplay.lvclass">)  [unwired: 7 in]
              }
              event "MAX FEEDRATE.Config_SetFeedrate": Value Change {
                n119 = event-data() -> ("NewVal"=w318:bool)  [unwired: 1 in]
                n120 = call "CheckButtoneTrue.vi"("IN"=w318) -> ("OUT"=w315:bool)  [unwired: 10 in]
                n121 = Unbundle By Name("MAX FEEDRATE") -> ("DATA"=w306:cluster{"X":dbl, "Y":dbl, "Z":dbl})
                n122 = To Variant(anything=w306) -> (Variant=w309:variant)
                n123 = call-dynamic "initMcode.vi"("CheckMenu"=w315, "error in (no error)"=w312, "mCode"=SelectMcode."M203_SetMaxFeedRate", "DataVariant"=w309, "XuLyDataDisplay in"=w316) -> ("error out"=w311:errorcluster, "McodeOut"=w308:string, "XuLyDataDisplay out"=w317:refnum<class "XuLyDataDisplay.lvclass">)  [unwired: 4 in]
                n124 = call-dynamic "WriteDataToQueueCMD.vi"("error in (no error)"=w311, "DataIn"=w308, "ParameterConf in"=w317) -> ("error out"=w314:errorcluster, "ParameterConf out"=w313:refnum<class "XuLyDataDisplay.lvclass">)  [unwired: 7 in]
              }
              event "MAX ACCEL.Config_SetMaxACCEL": Value Change {
                n125 = event-data() -> ("NewVal"=w331:bool)  [unwired: 1 in]
                n126 = call "CheckButtoneTrue.vi"("IN"=w331) -> ("OUT"=w330:bool)  [unwired: 10 in]
                n127 = Unbundle By Name("MAX ACCEL") -> ("DATA"=w320:cluster{"X":dbl, "Y":dbl, "Z":dbl})
                n128 = To Variant(anything=w320) -> (Variant=w322:variant)
                n129 = call-dynamic "initMcode.vi"("CheckMenu"=w330, "error in (no error)"=w328, "mCode"=SelectMcode."M201_SetMaxACCEL", "DataVariant"=w322, "XuLyDataDisplay in"=w329) -> ("error out"=w325:errorcluster, "McodeOut"=w326:string, "XuLyDataDisplay out"=w327:refnum<class "XuLyDataDisplay.lvclass">)  [unwired: 4 in]
                n130 = call-dynamic "WriteDataToQueueCMD.vi"("error in (no error)"=w325, "DataIn"=w326, "ParameterConf in"=w327) -> ("error out"=w323:errorcluster, "ParameterConf out"=w324:refnum<class "XuLyDataDisplay.lvclass">)  [unwired: 7 in]
              }
              event "STEPSIZE.Config_SetStepSize": Value Change {
                n131 = event-data() -> ("NewVal"=w343:bool)  [unwired: 1 in]
                n132 = call "CheckButtoneTrue.vi"("IN"=w343) -> ("OUT"=w336:bool)  [unwired: 10 in]
                n133 = Unbundle By Name("STEPSIZE") -> ("DATA"=w334:cluster{"X":dbl, "Y":dbl, "Z":dbl})
                n134 = To Variant(anything=w334) -> (Variant=w335:variant)
                n135 = call-dynamic "initMcode.vi"("CheckMenu"=w336, "error in (no error)"=w337, "mCode"=SelectMcode."M92_SetAxisStepPerUnit", "DataVariant"=w335, "XuLyDataDisplay in"=w342) -> ("error out"=w338:errorcluster, "XuLyDataDisplay out"=w341:refnum<class "XuLyDataDisplay.lvclass">)  [unwired: 4 in, 1 out]
                n136 = call-dynamic "WriteDataToQueueCMD.vi"("error in (no error)"=w338, "ParameterConf in"=w341) -> ("error out"=w339:errorcluster, "ParameterConf out"=w340:refnum<class "XuLyDataDisplay.lvclass">)  [unwired: 8 in]
              }
              event "Config_SaveEEPROM": Value Change {
                n137 = event-data() -> ("NewVal"=w353:bool)  [unwired: 1 in]
                n138 = call "CheckButtoneTrue.vi"("IN"=w353) -> ("OUT"=w346:bool)  [unwired: 10 in]
                n139 = call-dynamic "initMcode.vi"("CheckMenu"=w346, "error in (no error)"=w351, "mCode"=SelectMcode."M500_SaveEprom", "XuLyDataDisplay in"=w352) -> ("error out"=w347:errorcluster, "McodeOut"=w345:string, "XuLyDataDisplay out"=w350:refnum<class "XuLyDataDisplay.lvclass">)  [unwired: 5 in]
                n140 = call-dynamic "WriteDataToQueueCMD.vi"("error in (no error)"=w347, "DataIn"=w345, "ParameterConf in"=w350) -> ("error out"=w348:errorcluster, "ParameterConf out"=w349:refnum<class "XuLyDataDisplay.lvclass">)  [unwired: 7 in]
              }
              event "Send Gcode manual.SEND GCODE": Value Change {
                n141 = event-data() -> ()  [unwired: 1 in, 1 out]
                n142 = Unbundle By Name("Send Gcode manual") -> ("GCODE USET INPUT"=w363:string)
                n143 = call-dynamic "initGcode.vi"("gCode"=SelectGcode."sendGcodeString", "error in (no error)"=w364, "Gcode In"=w363, "XuLyDataDisplay in"=w366) -> ("error out"=w361:errorcluster, "GcodeString Out"=w358:string, "XuLyDataDisplay out"=w362:refnum<class "XuLyDataDisplay.lvclass">)  [unwired: 5 in]
                n144 = call-dynamic "WriteDataToQueueCMD.vi"("error in (no error)"=w361, "DataIn"=w358, "ParameterConf in"=w362) -> ("error out"=w359:errorcluster, "ParameterConf out"=w360:refnum<class "XuLyDataDisplay.lvclass">)  [unwired: 7 in]
                n145 = call-dynamic "ReadEmptyString.vi"("XuLyDataDisplay in"=w360) -> ("Boolean"=w356:bool, "String"=w355:string, "XuLyDataDisplay out"=w357:refnum<class "XuLyDataDisplay.lvclass">)  [unwired: 7 in, 1 out]
                n146 = Bundle("String"=w355, "Boolean"=w356) -> (w354:cluster{"String":string, "Boolean":bool})  [unwired: 1 in]
                n147 = property on="Send Gcode manual" class="Clust"("Val(Sgnl)"=w354) -> ()  [unwired: 2 in, 2 out]
              }
              event "Start Auto": Value Change {
                n148 = event-data() -> ("NewVal"=w371:bool)  [unwired: 1 in]
                n149 = global write "StartAutoandGcode.vi" "Start Auto"(w371) -> ()
                n150 = call "GCode File to Array.vi"("File Path"="File to Cut") -> ("G-Code Array"=w368:string[])  [unwired: 10 in]
                "G-Code Array 2" <- w368
                n151 = global write "StartAutoandGcode.vi" "G-Code Array 2"(w368) -> ()
              }
              event "Move.OK Button": Value Change {
                w387 = 0.0 ("X0")
                n152 = event-data() -> ()  [unwired: 1 in, 6 out]
                n153 = call-dynamic "Read PARA.vi"("error in (no error)"=w382, "ParameterConf in"=w383) -> ("error out"=w375:errorcluster, "ParameterConf out"=w381:refnum<class "XuLyDataDisplay.lvclass">)  [unwired: 6 in, 2 out]
                n154 = Unbundle By Name("Move") -> ("X"=w392:dbl, "Y"=w391:dbl)
                n155 = call "ScaraInverseKinematics.vi"("Y0"=w387, "X0"=w387, "L3"=w387, "L2"=23.0, "L1"=43.0, "Y"=w391, "X"=w392) -> ("angle 2"=w386:dbl, "angle 1"=w384:dbl)  [unwired: 3 in]
                n156 = Add(x=w384, y=w386) -> (x+y=w385:dbl)
                n157 = Bundle("angle 1"=w384, w385, 0) -> (w376:cluster{"angle 1":dbl, dbl, i32})  [unwired: 1 in]
                "output cluster 2" <- w376
                n158 = call-dynamic "initGcode.vi"("gCode"=SelectGcode."G1XY", "error in (no error)"=w375, "PosSetG92"=w376, "XuLyDataDisplay in"=w381) -> ("error out"=w379:errorcluster, "GcodeString Out"=w378:string, "XuLyDataDisplay out"=w380:refnum<class "XuLyDataDisplay.lvclass">)  [unwired: 5 in]
                n159 = call-dynamic "WriteDataToQueueCMD.vi"("error in (no error)"=w379, "DataIn"=w378, "ParameterConf in"=w380) -> ("error out"=w374:errorcluster, "ParameterConf out"=w373:refnum<class "XuLyDataDisplay.lvclass">)  [unwired: 7 in]
              }
              event "CONTROL PWM.WAIT PIN.PIN INPUT", "CONTROL PWM.FAN 3.PWM", "CONTROL PWM.FAN 2.PWM", "CONTROL PWM.FAN 1.PWM", "CONTROL PWM.SPIN.PWM", "PARA": Value Change {
                n160 = event-data() -> ()  [unwired: 1 in, 6 out]
              }
              event "BUTTON CONTROL MANUAL.Control_ButtonX-": Value Change {
                n161 = event-data() -> ("NewVal"=w406:bool)  [unwired: 1 in]
                n162 = call "CheckButtoneTrue.vi"("IN"=w406) -> ("OUT"=w399:bool)  [unwired: 10 in]
                n163 = call-dynamic "initGcode.vi"("Che Do"=w399, "gCode"=SelectGcode."JogX-", "error in (no error)"=w401, "XuLyDataDisplay in"=w402) -> ("error out"=w404:errorcluster, "GcodeString Out"=w398:string, "XuLyDataDisplay out"=w405:refnum<class "XuLyDataDisplay.lvclass">)  [unwired: 5 in]
                n164 = call-dynamic "WriteDataToQueueCMD.vi"("error in (no error)"=w404, "DataIn"=w398, "ParameterConf in"=w405) -> ("error out"=w400:errorcluster, "ParameterConf out"=w397:refnum<class "XuLyDataDisplay.lvclass">)  [unwired: 7 in]
              }
              event "CONTROL PWM.SOLENOID.AddFile_ButtonSolenoid": Value Change {
                n165 = event-data() -> ("NewVal"=w422:bool)  [unwired: 1 in]
                n166 = call "CheckButtoneTrue.vi"("IN"=w422) -> ("OUT"=w412:bool)  [unwired: 10 in]
                n167 = call-dynamic "ReadParameter.vi"("ParameterConf in"=w421, "error in (no error)"=w420, "Parameter"=T23."Solenoid") -> ("ParameterConf out"=w419:refnum<class "XuLyDataDisplay.lvclass">, "DataOutClust"=w410:T26, "error out"=w417:errorcluster)  [unwired: 4 in, 1 out]
                n168 = Unbundle By Name(w410) -> ("PWM"=w409:dbl)
                n169 = To Variant(anything=w409) -> (Variant=w414:variant)
                n170 = call-dynamic "initMcode.vi"("CheckMenu"=w412, "error in (no error)"=w417, "mCode"=SelectMcode."M380_381_SetSoleNoid_On_Off", "DataVariant"=w414, "XuLyDataDisplay in"=w419) -> ("error out"=w416:errorcluster, "McodeOut"=w413:string, "XuLyDataDisplay out"=w418:refnum<class "XuLyDataDisplay.lvclass">)  [unwired: 4 in]
                n171 = call-dynamic "InsetStringToFileGcode.vi"("error in (no error)"=w416, "StringFileGcode"=w413, "ParameterConf in"=w418) -> ("error out"=w407:errorcluster, "ParameterConf out"=w408:refnum<class "XuLyDataDisplay.lvclass">)  [unwired: 7 in]
              }
              event "CONTROL PWM.FAN 3.AddFile_ButtonFan3": Value Change {
                n172 = event-data() -> ("NewVal"=w437:bool)  [unwired: 1 in]
                n173 = call "CheckButtoneTrue.vi"("IN"=w437) -> ("OUT"=w428:bool)  [unwired: 10 in]
                n174 = call-dynamic "ReadParameter.vi"("ParameterConf in"=w436, "error in (no error)"=w435, "Parameter"=T23."Fan3") -> ("ParameterConf out"=w434:refnum<class "XuLyDataDisplay.lvclass">, "DataOutClust"=w426:T26, "error out"=w433:errorcluster)  [unwired: 4 in, 1 out]
                n175 = Unbundle By Name(w426) -> ("PWM"=w425:dbl)
                n176 = call-dynamic "initMcode.vi"("CheckMenu"=w428, "error in (no error)"=w433, "mCode"=SelectMcode."M106_SetFan3", "DataVariant"=w425, "XuLyDataDisplay in"=w434) -> ("error out"=w431:errorcluster, "McodeOut"=w430:string, "XuLyDataDisplay out"=w432:refnum<class "XuLyDataDisplay.lvclass">)  [unwired: 4 in]
                n177 = call-dynamic "InsetStringToFileGcode.vi"("error in (no error)"=w431, "StringFileGcode"=w430, "ParameterConf in"=w432) -> ("error out"=w423:errorcluster, "ParameterConf out"=w424:refnum<class "XuLyDataDisplay.lvclass">)  [unwired: 7 in]
              }
              event "CONTROL PWM.FAN 2.AddFile_ButtonFan2": Value Change {
                n178 = event-data() -> ("NewVal"=w452:bool)  [unwired: 1 in]
                n179 = call-dynamic "ReadParameter.vi"("ParameterConf in"=w447, "error in (no error)"=w446, "Parameter"=T23."Fan2") -> ("ParameterConf out"=w451:refnum<class "XuLyDataDisplay.lvclass">, "DataOutClust"=w441:T26, "error out"=w450:errorcluster)  [unwired: 4 in, 1 out]
                n180 = call "CheckButtoneTrue.vi"("IN"=w452) -> ("OUT"=w443:bool)  [unwired: 10 in]
                n181 = Unbundle By Name(w441) -> ("PWM"=w440:dbl)
                n182 = call-dynamic "initMcode.vi"("CheckMenu"=w443, "error in (no error)"=w450, "mCode"=SelectMcode."M106_SetFan2", "DataVariant"=w440, "XuLyDataDisplay in"=w451) -> ("error out"=w448:errorcluster, "McodeOut"=w445:string, "XuLyDataDisplay out"=w449:refnum<class "XuLyDataDisplay.lvclass">)  [unwired: 4 in]
                n183 = call-dynamic "InsetStringToFileGcode.vi"("error in (no error)"=w448, "StringFileGcode"=w445, "ParameterConf in"=w449) -> ("error out"=w438:errorcluster, "ParameterConf out"=w439:refnum<class "XuLyDataDisplay.lvclass">)  [unwired: 7 in]
              }
              event "CONTROL PWM.FAN 1.AddFile_ButtonFan1": Value Change {
                n184 = event-data() -> ("NewVal"=w465:bool)  [unwired: 1 in]
                n185 = call-dynamic "Read FAN1.vi"("error in (no error)"=w463, "ParameterConf in"=w464) -> ("error out"=w461:errorcluster, "FAN1"=w457:dbl, "ParameterConf out"=w460:refnum<class "XuLyDataDisplay.lvclass">)  [unwired: 6 in, 1 out]
                n186 = call "CheckButtoneTrue.vi"("IN"=w465) -> ("OUT"=w455:bool)  [unwired: 10 in]
                n187 = call-dynamic "initMcode.vi"("CheckMenu"=w455, "error in (no error)"=w461, "mCode"=SelectMcode."M106_SetFan1", "DataVariant"=w457, "XuLyDataDisplay in"=w460) -> ("error out"=w462:errorcluster, "McodeOut"=w458:string, "XuLyDataDisplay out"=w459:refnum<class "XuLyDataDisplay.lvclass">)  [unwired: 4 in]
                n188 = call-dynamic "InsetStringToFileGcode.vi"("error in (no error)"=w462, "StringFileGcode"=w458, "ParameterConf in"=w459) -> ("error out"=w453:errorcluster, "ParameterConf out"=w454:refnum<class "XuLyDataDisplay.lvclass">)  [unwired: 7 in]
              }
              event "CONTROL PWM.SPIN.ButtonSPINDLE_ADD_FILE": Value Change {
                n189 = event-data() -> ("NewVal"=w480:bool)  [unwired: 1 in]
                n190 = call "CheckButtoneTrue.vi"("IN"=w480) -> ("OUT"=w471:bool)  [unwired: 10 in]
                n191 = call-dynamic "ReadParameter.vi"("ParameterConf in"=w479, "error in (no error)"=w478, "Parameter"=T23."Spindle") -> ("ParameterConf out"=w476:refnum<class "XuLyDataDisplay.lvclass">, "DataOutClust"=w469:T26, "error out"=w475:errorcluster)  [unwired: 4 in, 1 out]
                n192 = Unbundle By Name(w469) -> ("PWM"=w468:dbl)
                n193 = call-dynamic "initMcode.vi"("CheckMenu"=w471, "error in (no error)"=w475, "mCode"=SelectMcode."M3_SetSpindle", "DataVariant"=w468, "XuLyDataDisplay in"=w476) -> ("error out"=w474:errorcluster, "McodeOut"=w473:string, "XuLyDataDisplay out"=w477:refnum<class "XuLyDataDisplay.lvclass">)  [unwired: 4 in]
                n194 = call-dynamic "InsetStringToFileGcode.vi"("error in (no error)"=w474, "StringFileGcode"=w473, "ParameterConf in"=w477) -> ("error out"=w466:errorcluster, "ParameterConf out"=w467:refnum<class "XuLyDataDisplay.lvclass">)  [unwired: 7 in]
              }
              event "BUTTON CONTROL GCODE FILE.FILE.AddFile_ButtonDeleteLastLine": Value Change {
                n195 = event-data() -> ("NewVal"=w486:bool)  [unwired: 1 in]
                n196 = call "CheckButtoneTrue.vi"("IN"=w486) -> ("OUT"=w483:bool)  [unwired: 10 in]
                n197 = call-dynamic "deleteLastLine.vi"("TypeControl"=w483, "error in (no error)"=w484, "XuLyDataDisplay in"=w485) -> ("error out"=w481:errorcluster, "XuLyDataDisplay out"=w482:refnum<class "XuLyDataDisplay.lvclass">)  [unwired: 7 in]
              }
              event "CONTROL PWM.WAIT PIN.Control_ButtonWaitPin": Value Change {
                n198 = event-data() -> ()  [unwired: 1 in, 1 out]
              }
              event "BUTTON CONTROL GCODE FILE.FILE.AddFile_ButtonDeleteAll": Value Change {
                n199 = event-data() -> ()  [unwired: 1 in, 1 out]
                n200 = call-dynamic "Write StringFileGcode.vi"("error in (no error)"=w490, "StringFileGcode"="", "ParameterConf in"=w493) -> ("error out"=w491:errorcluster, "ParameterConf out"=w489:refnum<class "XuLyDataDisplay.lvclass">)  [unwired: 7 in]
              }
              event "BUTTON CONTROL GCODE FILE.MOTION.AddFile_ButtonGoHome": Value Change {
                n201 = event-data() -> ("NewVal"=w503:bool)  [unwired: 1 in]
                n202 = call "CheckButtoneTrue.vi"("IN"=w503) -> ("OUT"=w496:bool)  [unwired: 10 in]
                n203 = call-dynamic "initGcode.vi"("Che Do"=w496, "gCode"=SelectGcode."G28AutoHome", "error in (no error)"=w499, "XuLyDataDisplay in"=w501) -> ("error out"=w498:errorcluster, "GcodeString Out"=w495:string, "XuLyDataDisplay out"=w500:refnum<class "XuLyDataDisplay.lvclass">)  [unwired: 5 in]
                n204 = call-dynamic "InsetStringToFileGcode.vi"("error in (no error)"=w498, "StringFileGcode"=w495, "ParameterConf in"=w500) -> ("error out"=w502:errorcluster, "ParameterConf out"=w494:refnum<class "XuLyDataDisplay.lvclass">)  [unwired: 7 in]
              }
              event "BUTTON CONTROL GCODE FILE.FILE.AddFile_ButtonSaveFile": Value Change {
                n205 = event-data() -> ("NewVal"=w513:bool)  [unwired: 1 in]
                n206 = call "CheckButtoneTrue.vi"("IN"=w513) -> ("OUT"=w504:bool)  [unwired: 10 in]
                n207 = call-dynamic "Read StringFileGcode.vi"("error in (no error)"=w511, "ParameterConf in"=w512) -> ("error out"=w507:errorcluster, "StringFileGcode"=w509:string, "ParameterConf out"=w510:refnum<class "XuLyDataDisplay.lvclass">)  [unwired: 7 in]
                n208 = call-dynamic "SaveFile.vi"("TyprControl"=w504, "error in (no error)"=w507, "text"=w509, "file path (use dialog)"="Link Save File", "XuLyDataDisplay in"=w510) -> ("error out"=w505:errorcluster, "XuLyDataDisplay out"=w506:refnum<class "XuLyDataDisplay.lvclass">)  [unwired: 5 in]
              }
              event "BUTTON CONTROL GCODE FILE.MOTION.AddFile_ButtonAddG1": Value Change {
                n209 = event-data() -> ("NewVal"=w525:bool)  [unwired: 1 in]
                n210 = call-dynamic "Read PARA.vi"("error in (no error)"=w521, "ParameterConf in"=w524) -> ("error out"=w518:errorcluster, "ParameterConf out"=w520:refnum<class "XuLyDataDisplay.lvclass">)  [unwired: 6 in, 2 out]
                n211 = call "CheckButtoneTrue.vi"("IN"=w525) -> ("OUT"=w516:bool)  [unwired: 10 in]
                n212 = call-dynamic "initGcode.vi"("Che Do"=w516, "gCode"=SelectGcode."G1LinearMove", "error in (no error)"=w518, "XuLyDataDisplay in"=w520) -> ("error out"=w517:errorcluster, "GcodeString Out"=w514:string, "XuLyDataDisplay out"=w519:refnum<class "XuLyDataDisplay.lvclass">)  [unwired: 5 in]
                n213 = call-dynamic "InsetStringToFileGcode.vi"("error in (no error)"=w517, "StringFileGcode"=w514, "ParameterConf in"=w519) -> ("error out"=w522:errorcluster, "ParameterConf out"=w523:refnum<class "XuLyDataDisplay.lvclass">)  [unwired: 7 in]
              }
              event "BUTTON CONTROL GCODE FILE.MOTION.AddFile_ButtonAddG0": Value Change {
                n214 = event-data() -> ("NewVal"=w535:bool)  [unwired: 1 in]
                n215 = call "CheckButtoneTrue.vi"("IN"=w535) -> ("OUT"=w528:bool)  [unwired: 10 in]
                n216 = call-dynamic "initGcode.vi"("Che Do"=w528, "gCode"=SelectGcode."G0LinearMove", "error in (no error)"=w533, "XuLyDataDisplay in"=w534) -> ("error out"=w529:errorcluster, "GcodeString Out"=w526:string, "XuLyDataDisplay out"=w530:refnum<class "XuLyDataDisplay.lvclass">)  [unwired: 5 in]
                n217 = call-dynamic "InsetStringToFileGcode.vi"("error in (no error)"=w529, "StringFileGcode"=w526, "ParameterConf in"=w530) -> ("error out"=w531:errorcluster, "ParameterConf out"=w532:refnum<class "XuLyDataDisplay.lvclass">)  [unwired: 7 in]
              }
              event "BUTTON CONTROL MANUAL.Control_ButtonZ+": Value Change {
                n218 = event-data() -> ("NewVal"=w546:bool)  [unwired: 1 in]
                n219 = call "CheckButtoneTrue.vi"("IN"=w546) -> ("OUT"=w543:bool)  [unwired: 10 in]
                n220 = call-dynamic "initGcode.vi"("Che Do"=w543, "gCode"=SelectGcode."JogZ+", "error in (no error)"=w544, "XuLyDataDisplay in"=w545) -> ("error out"=w539:errorcluster, "GcodeString Out"=w537:string, "XuLyDataDisplay out"=w542:refnum<class "XuLyDataDisplay.lvclass">)  [unwired: 5 in]
                n221 = call-dynamic "WriteDataToQueueCMD.vi"("error in (no error)"=w539, "DataIn"=w537, "ParameterConf in"=w542) -> ("error out"=w540:errorcluster, "ParameterConf out"=w541:refnum<class "XuLyDataDisplay.lvclass">)  [unwired: 7 in]
              }
              event "BUTTON CONTROL MANUAL.Control_ButtonY+": Value Change {
                n222 = event-data() -> ("NewVal"=w556:bool)  [unwired: 1 in]
                n223 = call "CheckButtoneTrue.vi"("IN"=w556) -> ("OUT"=w553:bool)  [unwired: 10 in]
                n224 = call-dynamic "initGcode.vi"("Che Do"=w553, "gCode"=SelectGcode."JogY+", "error in (no error)"=w554, "XuLyDataDisplay in"=w555) -> ("error out"=w550:errorcluster, "GcodeString Out"=w551:string, "XuLyDataDisplay out"=w552:refnum<class "XuLyDataDisplay.lvclass">)  [unwired: 5 in]
                n225 = call-dynamic "WriteDataToQueueCMD.vi"("error in (no error)"=w550, "DataIn"=w551, "ParameterConf in"=w552) -> ("error out"=w547:errorcluster, "ParameterConf out"=w548:refnum<class "XuLyDataDisplay.lvclass">)  [unwired: 7 in]
              }
              event "BUTTON CONTROL MANUAL.Control_ButtonY-": Value Change {
                n226 = event-data() -> ("NewVal"=w566:bool)  [unwired: 1 in]
                n227 = call "CheckButtoneTrue.vi"("IN"=w566) -> ("OUT"=w559:bool)  [unwired: 10 in]
                n228 = call-dynamic "initGcode.vi"("Che Do"=w559, "gCode"=SelectGcode."JogY-", "error in (no error)"=w560, "XuLyDataDisplay in"=w561) -> ("error out"=w563:errorcluster, "GcodeString Out"=w564:string, "XuLyDataDisplay out"=w565:refnum<class "XuLyDataDisplay.lvclass">)  [unwired: 5 in]
                n229 = call-dynamic "WriteDataToQueueCMD.vi"("error in (no error)"=w563, "DataIn"=w564, "ParameterConf in"=w565) -> ("error out"=w557:errorcluster, "ParameterConf out"=w558:refnum<class "XuLyDataDisplay.lvclass">)  [unwired: 7 in]
              }
              event "BUTTON CONTROL MANUAL.Control_ButtonZ-": Value Change {
                n230 = event-data() -> ("NewVal"=w576:bool)  [unwired: 1 in]
                n231 = call "CheckButtoneTrue.vi"("IN"=w576) -> ("OUT"=w568:bool)  [unwired: 10 in]
                n232 = call-dynamic "initGcode.vi"("Che Do"=w568, "gCode"=SelectGcode."JogZ-", "error in (no error)"=w570, "XuLyDataDisplay in"=w571) -> ("error out"=w573:errorcluster, "GcodeString Out"=w574:string, "XuLyDataDisplay out"=w575:refnum<class "XuLyDataDisplay.lvclass">)  [unwired: 5 in]
                n233 = call-dynamic "WriteDataToQueueCMD.vi"("error in (no error)"=w573, "DataIn"=w574, "ParameterConf in"=w575) -> ("error out"=w569:errorcluster, "ParameterConf out"=w567:refnum<class "XuLyDataDisplay.lvclass">)  [unwired: 7 in]
              }
            }
          }
          frame "End" {
          }
          frame "writeGlobal" {
            n234 = Unbundle By Name("CONTROL PWM") -> ("SPIN.PWM"=w599:dbl, "FAN 2.PWM"=w598:dbl, "FAN 1.PWM"=w597:dbl, "FAN 3.PWM"=w596:dbl, "WAIT PIN.PIN INPUT"=w595:dbl, "SOLENOID.Control_ButtonSolenoid"=w594:bool)
            n235 = Unbundle By Name("PARA") -> ("STEP"=w586:i16, "FEEDRATE"=w585:dbl)
            n236 = Bundle By Name(cluster=cluster{"STEP":i16, "FEEDRATE":dbl} {"STEP"=0, "FEEDRATE"=0.0} ("PARA"), "STEP"=w586, "FEEDRATE"=w585) -> (w583:cluster{"STEP":i16, "FEEDRATE":dbl})
            n237 = Bundle By Name(cluster=T25 {"SPIN"=0.0, "FAN2"=0.0, "FAN1"=0.0, "FAN3"=0.0, "WAIT PIN "=0.0} ("CONTROL PWM"), "SPIN"=w599, "FAN2"=w598, "FAN1"=w597, "FAN3"=w596, "WAIT PIN"=w595) -> (w602:T25)
            n238 = call-dynamic "Updatevalue.vi"("ParameterConf in"=w593, "CONTROL PWM"=w602, "PARA"=w583, "error in (no error)"=w592) -> ("ParameterConf out"=w601:refnum<class "XuLyDataDisplay.lvclass">, "error out"=w600:errorcluster)  [unwired: 5 in]
            n239 = call-dynamic "UpdateSoleNoid.vi"("error in (no error)"=w600, "Boolean"=w594, "ParameterConf in"=w601) -> ("error out"=w590:errorcluster, "ParameterConf out"=w591:refnum<class "XuLyDataDisplay.lvclass">)  [unwired: 7 in]
          }
          frame "schedules500ms" {
            n240 = global read "StartAutoandGcode.vi" "StateModeSoftWare"() -> (→"statusMode":T2)
            n241 = call-dynamic "Read StringFileGcode.vi"("error in (no error)"=w609, "ParameterConf in"=w610) -> ("error out"=w606:errorcluster, "StringFileGcode"=→"GCODE ADD":string, "ParameterConf out"=w607:refnum<class "XuLyDataDisplay.lvclass">)  [unwired: 7 in]
          }
        }
        n242 = node-c288() -> ()  [unwired: 1 in, 1 out]
        n243 = call-dynamic "Write StateDisplay.vi"("error in (no error)"=w48, "StateDisplay"=w46, "ParameterConf in"=w45) -> ("error out"=w49:errorcluster, "ParameterConf out"=w50:refnum<class "XuLyDataDisplay.lvclass">)  [unwired: 7 in]
      }
      n244 = node-c288(w39) -> ()  [unwired: 1 out]
    }
  }
  n245 = Obtain Queue(name (unnamed)=w23, element data type=w23) -> (queue out=w19:refnum<queue>, error out=w7:errorcluster)  [unwired: 3 in, 1 out]
  n246 = Obtain Queue(element data type=T15 {"Command"=enum."updatePos", "POS"={"X"=0.0, "Y"=0.0, "Z"=0.0}, "DEGREES"={"X"=0.0, "Y"=0.0}}, error in (no error)=w7) -> (queue out=w8:refnum<queue>, error out=w17:errorcluster)  [unwired: 3 in, 1 out]
  n247 = Merge Errors(w17, w21, w22) -> (w13:errorcluster)
  n248 = Bundle(cluster=T16 {"Serial Data Gcode"=refnum, "cmdUpdateDisplay"=refnum}, "Serial Data Gcode"=w19, "cmdUpdateDisplay"=w8) -> (w14:T16)
  n249 = Bundle("cluster"=w14, "error IO"=w13) -> (w11:cluster{"cluster":T16, "error IO":errorcluster})  [unwired: 1 in]
  n250 = Unbundle By Name(w11) -> ("cluster"=w12:T16, "error IO"=w5:errorcluster)
  n251 = call "mainControlSerial.vi"("error in (no error)"=w5, "Queue In"=w12) -> ("error out"=w6:errorcluster)  [unwired: 9 in]
  n252 = call "mainControlAuto.vi"("error IO"=w5, "QueueCluste"=w12) -> ("error IO 2"=w16:errorcluster)  [unwired: 9 in]
  n253 = while {
    tunnel: w11 -> [_]
    shift-right: [w614] -> _
    shift-left: w9 -> [w620]
    shift-right: [w616] -> _
    shift-left: Robot_testing_instructions."Init 1 - Application" -> [w617]
    stop <- w618 stop-if-true
    n254 = case shown="\"Draw Robot\"" w617 {
      selector: w617 -> [_ _ _ w646 w649 w651 _]
      tunnel: w620 -> [w622 w623 w638 w647 w648 w650 w666]
      tunnel: [w622 w626 w637 w647 w648 w650 w665] -> w614
      tunnel: [Robot_testing_instructions."Error Handling" Robot_testing_instructions."Calculates" Robot_testing_instructions."Draw Robot" w646 w649 w651 Robot_testing_instructions."Calculates"] -> w616
      frame "idle", Default {
      }
      frame "Draw Robot" {
        n255 = Unbundle By Name(w623) -> ("Robot Definition"=w634:T12)
        n256 = call "Create Robot State Machine.vi"("Robot Definition"=w634) -> ("error out"=→"error out 2":errorcluster, "Cluster"=w633:T27)  [unwired: 9 in]
        n257 = Unbundle By Name(w633) -> ("Scene ref"=w627:refnum<vi>, "Sand box ref"=w628:refnum<vi>, "Arm 1 ref"=w629:refnum<vi>, "Arm 1 Offset"=w630:cluster{"X":sgl, "Y":sgl, "Z":sgl}[], "Arm 2 ref"=w631:refnum<vi>, "Arm 2 Offset"=w632:cluster{"X":sgl, "Y":sgl, "Z":sgl}[])
        n258 = Bundle By Name(cluster=w623, "Scene ref"=w627, "sand box"=w628, "Arm 1 ref"=w629, "Arm 1 offset"=w630, "Arm 2 ref"=w631, "Arm 2 offset"=w632) -> (w626:T13)
      }
      frame "Init 1 - Application" {
        n259 = Bundle By Name(cluster=w638, "Robot Definition.Base"=sgl 4.0, "Robot Definition.L1"=sgl 4.3, "Robot Definition.L2"=sgl 2.3, "Robot Definition.L3"=sgl 0.0, "Robot Definition.X0"=sgl 0.0, "Robot Definition.Z0"=sgl 0.0, "A1"=0.0, "A2"=0.0) -> (w637:T13)
      }
      frame "Quit" {
      }
      frame "Close" {
      }
      frame "Error Handling" {
      }
      frame "Calculates" {
        n260 = Unbundle By Name(w666) -> ("Arm 2 offset"=w680:cluster{"X":sgl, "Y":sgl, "Z":sgl}[], "Arm 2 ref"=w670:refnum<vi>, "Arm 1 offset"=w677:cluster{"X":sgl, "Y":sgl, "Z":sgl}[], "Arm 1 ref"=w674:refnum<vi>)
        n261 = local read "degrees"() -> (w655:cluster{"A":dbl, "B":dbl})
        n262 = Index Array(array=w677) -> (element #1=w673:cluster{"X":sgl, "Y":sgl, "Z":sgl}, element #2=w671:cluster{"X":sgl, "Y":sgl, "Z":sgl})  [unwired: 2 in]
        n263 = call <vilib>:"Clear Transformation.vi"("Object Refnum In"=w674) -> ("error out"=w664:errorcluster, "Object Refnum Out"=w679:refnum<vi>)  [unwired: 9 in]
        n264 = call <vilib>:"Set Translation.vi"("error in (no error)"=w664, "Translation"=w673, "Scene Object"=w679) -> ("error out"=w663:errorcluster, "Translated Object"=w675:refnum<vi>)  [unwired: 7 in]
        n265 = Unbundle By Name(w655) -> ("A"=w653:dbl, "B"=w654:dbl)
        n266 = call <vilib>:"Rotate Y-axis.vi"("Relative?"=TRUE, "error in (no error)"=w663, "angle"=w653, "Scene Object In"=w675) -> ("error out"=w662:errorcluster, "Scene Object Out"=w678:refnum<vi>)  [unwired: 6 in]
        n267 = call <vilib>:"Translate Object.vi"("error in (no error)"=w662, "Translation"=w671, "Scene.Object In"=w678) -> ("error out"=w661:errorcluster, "Scene.Object Out"=w676:refnum<vi>)  [unwired: 7 in]
        n268 = Subtract(x=w654, y=w653) -> (x-y=w652:dbl)
        n269 = call <vilib>:"Clear Transformation.vi"("error in (no error)"=w661, "Object Refnum In"=w670) -> ("error out"=w660:errorcluster, "Object Refnum Out"=w683:refnum<vi>)  [unwired: 8 in]
        n270 = Index Array(array=w680) -> (element #1=w669:cluster{"X":sgl, "Y":sgl, "Z":sgl}, element #2=w667:cluster{"X":sgl, "Y":sgl, "Z":sgl})  [unwired: 2 in]
        n271 = call <vilib>:"Set Translation.vi"("error in (no error)"=w660, "Translation"=w669, "Scene Object"=w683) -> ("error out"=w659:errorcluster, "Translated Object"=w684:refnum<vi>)  [unwired: 7 in]
        n272 = call <vilib>:"Rotate Y-axis.vi"("Relative?"=TRUE, "error in (no error)"=w659, "angle"=w652, "Scene Object In"=w684) -> ("error out"=w658:errorcluster, "Scene Object Out"=w682:refnum<vi>)  [unwired: 6 in]
        n273 = call <vilib>:"Translate Object.vi"("error in (no error)"=w658, "Translation"=w667, "Scene.Object In"=w682) -> ("error out"=→"error out":errorcluster, "Scene.Object Out"=w681:refnum<vi>)  [unwired: 7 in]
        n274 = Bundle By Name(cluster=w666, "Arm 1 ref"=w676, "Arm 2 ref"=w681) -> (w665:T13)
      }
    }
    n275 = Wait (ms)(milliseconds to wait=u32 10) -> ()  [unwired: 1 out]
    n276 = global read "StartAutoandGcode.vi" "EMG"() -> (w618:bool)
    n277 = Unbundle By Name(w614) -> ("Scene ref"=→"3D Picture":refnum<vi>)
  }
  n278 = Bundle("error out"=w6, "error IO 2"=w16) -> (w15:T28)  [unwired: 1 in]
  n279 = call-dynamic "Release Queue.vi"("error in (no error)"=w3, "ParameterConf in"=w4) -> ("error out"=w2:errorcluster)  [unwired: 8 in, 1 out]
  n280 = Unregister For Events(event registration refnum=w1) -> ()  [unwired: 1 in, 1 out]
  n281 = Bundle(w15, "error out"=w2) -> ()  [unwired: 1 in, 1 out]
